vi "test_F9P_fgv-ver.vi"() -> ()   [LabVIEW 2019] (continued)
N,0.221,K,A*35\r\n$GNGGA,065002.00,3723.57089,N,12657.01324,E,1,12,0.74,36.5,M,18.5,M,,*7A\r\n$GNGSA,A,3,17,19,06,12,05,02,09,,,,,,1.34,0.74,1.12,1*03\r\n$GNGSA,A,3,85,71,72,,,,,,,,,,1.34,0.74,1.12,2*0B\r\n$GNGSA,A,3,36,11,04,09,12,,,,,,,,1.34,0.74,1.12,3*0F\r\n$GNGSA,A,3,28,11,14,13,33,08,10,,,,,,1.34,0.74,1.12,4*07\r\n$GPGSV,4,1,13,02,67,338,32,04,06,036,14,05,50,265,42,06,56,081,36,1*65\r\n$GPGSV,4,2,13,07,08,102,,09,36,055,32,12,17,260,32,13,11,191,26,1*6E\r\n$GPGSV,4,3,13,17,16,158,36,19,34,162,29,25,11,291,25,29,09,322,26,1*67\r\n$GPGSV,4,4,13,30,03,132,,1*56\r\n$GPGSV,4,1,13,02,67,338,,04,06,036,,05,50,265,32,06,56,081,30,6*67\r\n$GPGSV,4,2,13,07,08,102,,09,36,055,39,12,17,260,20,13,11,191,,6*65\r\n$GPGSV,4,3,13,17,16,158,34,19,34,162,,25,11,291,20,29,09,322,26,6*6C\r\n$GPGSV,4,4,13,30,03,132,,6*51\r\n$GLGSV,2,1,06,70,51,030,,71,72,230,37,72,20,218,41,84,06,136,10,1*7D\r\n$GLGSV,2,2,06,85,61,118,37,86,55,338,,1*7E\r\n$GLGSV,2,1,06,70,51,030,,71,72,230,26,72,20,218,26,84,06,136,07,3*78\r\n$GLGSV,2,2,06,85,61,118,25,86,55,338,,3*7F\r\n$GAGSV,3,1,09,02,03,285,10,04,67,079,31,05,00,212,,09,47,197,38,7*74\r\n$GAGSV,3,2,09,11,78,050,27,12,30,117,31,18,58,277,45,19,15,041,,7*7F\r\n$GAGSV,3,3,09,36,37,315,22,7*4C\r\n$GAGSV,3,1,09,02,03,285,,04,67,079,34,05,00,212,,09,47,197,36,2*7B\r\n$GAGSV,3,2,09,11,78,050,27,12,30,117,31,18,58,277,35,19,15,041,,2*7D\r\n$GAGSV,3,3,09,36,37,315,34,2*4E\r\n$GBGSV,5,1,17,01,42,153,,03,45,207,,04,35,133,,05,09,257,,1*7C\r\n$GBGSV,5,2,17,06,29,183,,07,08,201,,08,66,357,29,09,08,194,,1*73\r\n$GBGSV,5,3,17,10,14,222,26,11,34,144,26,13,50,316,32,14,73,036,35,1*76\r\n$GBGSV,5,4,17,16,25,186,34,27,10,317,,28,61,307,30,33,75,247,37,1*75\r\n$GBGSV,5,5,17,34,10,143,,1*40\r\n$GBGSV,5,1,17,01,42,153,,03,45,207,,04,35,133,,05,09,257,,3*7E\r\n$GBGSV,5,2,17,06,29,183,,07,08,201,,08,66,357,21,09,08,194,,3*79\r\n$GBGSV,5,3,17,10,14,222,39,11,34,144,39,13,50,316,24,14,73,036,29,3*7E\r\n$GBGSV,5,4,17,16,25,186,33,27,10,317,,28,61,307,,33,75,247,,3*77\r\n$GBGSV,5,5,17,34,10,143,,3*42\r\n$GNGLL,3723.57089,N,12657.01324,E,065002.00,A,A*73\r\n$GNRMC,065003.00,A,3723.57090,N,12657.01323,E,0.098,,250720,,,A,V*1D\r\n$GNVTG,,T,,M,0.098,N,0.182,K,A*37\r\n$GNGGA,065003.00,3723.57090,N,12657.01323,E,1,12,0.74,36.5,M,18.5,M,,*74\r\n$GNGSA,A,3,17,19,06,12,05,02,09,,,,,,1.34,0.74,1.12,1*03\r\n$GNGSA,A,3,85,71,72,,,,,,,,,,1.34,0.74,1.12,2*0B\r\n$GNGSA,A,3,36,11,04,09,12,,,,,,,,1.34,0.74,1.12,3*0F\r\n$GNGSA,A,3,28,11,14,13,33,08,10,,,,,,1.34,0.74,1.12,4*07\r\n$GPGSV,4,1,13,02,67,338,34,04,06,036,09,05,50,265,43,06,56,081,33,1*6B\r\n$GPGSV,4,2,13,07,08,102,14,09,36,055,31,12,17,260,25,13,11,191,27,1*6F\r\n$GPGSV,4,3,13,17,16,158,35,19,34,162,27,25,11,291,20,29,09,322,23,1*6A\r\n$GPGSV,4,4,13,30,03,132,,1*56\r\n$GPGSV,4,1,13,02,67,338,,04,06,036,,05,50,265,32,06,56,081,21,6*67\r\n$GPGSV,4,2,13,07,08,102,,09,36,055,38,12,17,260,20,13,11,191,,6*64\r\n$GPGSV,4,3,13,17,16,158,36,19,34,162,,25,11,291,19,29,09,322,25,6*67\r\n$GPGSV,4,4,13,30,03,132,,6*51\r\n$GLGSV,2,1,06,70,51,030,,71,72,230,40,72,20,218,40,84,06,136,11,1*7D\r\n$GLGSV,2,2,06,85,61,118,37,86,55,338,,1*7E\r\n$GLGSV,2,1,06,70,51,030,,71,72,230,23,72,20,218,27,84,06,136,08,3*73\r\n$GLGSV,2,2,06,85,61,118,23,86,55,338,,3*79\r\n$GAGSV,3,1,09,02,03,285,08,04,67,079,25,05,00,212,,09,47,197,37,7*77\r\n$GAGSV,3,2,09,11,78,050,27,12,30,117,30,18,58,277,44,19,15,041,19,7*77\r\n$GAGSV,3,3,09,36,37,315,17,7*4A\r\n$GAGSV,3,1,09,02,03,285,,04,67,079,30,05,00,212,,09,47,197,33,2*7A\r\n$GAGSV,3,2,09,11,78,050,23,12,30,117,29,18,58,277,32,19,15,041,,2*77\r\n$GAGSV,3,3,09,36,37,315,34,2*4E\r\n$GBGSV,5,1,17,01,42,153,,03,45,207,,04,35,133,,05,09,257,,1*7C\r\n$GBGSV,5,2,17,06,29,183,,07,08,201,,08,66,357,28,09,08,194,,1*72\r\n$GBGSV,5,3,17,10,14,222,25,11,34,144,30,13,50,316,25,14,73,036,34,1*75\r\n$GBGSV,5,4,17,16,25,186,31,27,10,317,,28,61,307,30,33,75,247,39,1*7E\r\n$GBGSV,5,5,17,34,10,143,,1*40\r\n$GBGSV,5,1,17,01,42,153,,03,45,207,,04,35,133,,05,09,257,,3*7E\r\n$GBGSV,5,2,17,06,29,183,,07,08,201,,08,66,357,21,09,08,194,,3*79\r\n$GBGSV,5,3,17,10,14,222,39,11,34,144,41,13,50,316,25,14,73,036,28,3*71\r\n$GBGSV,5,4,17,16,25,186,33,27,10,317,,28,61,307,,33,75,247,,3*77\r\n$GBGSV,5,5,17,34,10,143,,3*42\r\n$GNGLL,3723.57090,N,12657.01323,E,065003.00,A,A*7D\r\n$GNRMC,065004.00,A,3723.57091,N,12657.01321,E,0.157,,250720,,,A,V*1B\r\n$GNVTG,,T,,M,0.157,N,0.291,K,A*34\r\n$GNGGA,065004.00,3723.57091,N,12657.01321,E,1,12,0.71,36.5,M,18.5,M,,*75\r\n$GNGSA,A,3,17,19,06,12,05,02,09,,,,,,1.26,0.71,1.04,1*02\r\n$GNGSA,A,3,85,71,72,,,,,,,,,,1.26,0.71,1.04,2*0A\r\n$GNGSA,A,3,36,11,04,09,12,,,,,,,,1.26,0.71,1.04,3*0E\r\n$GNGSA,A,3,28,11,14,13,33,08,10,,,,,,1.26,0.71,1.04,4*06\r\n$GPGSV,4,1,13,02,67,338,23,04,06,036,09,05,50,265,42,06,56,081,29,1*67\r\n$GPGSV,4,2,13,07,08,102,11,09,36,055,33,12,17,260,26,13,11,191,28,1*64\r\n$GPGSV,4,3,13,17,16,158,43,19,34,162,35,25,11,291,21,29,09,322,25,1*6F\r\n$GPGSV,4,4,13,30,03,132,,1*56\r\n$GPGSV,4,1,13,02,67,338,,04,06,036,,05,50,265,30,06,56,081,25,6*61\r\n$GPGSV,4,2,13,07,08,102,,09,36,055,37,12,17,260,20,13,11,191,,6*6B\r\n$GPGSV,4,3,13,17,16,158,32,19,34,162,,25,11,291,17,29,09,322,24,6*6C\r\n$GPGSV,4,4,13,30,03,132,,6*51\r\n$GLGSV,2,1,06,70,50,030,,71,72,230,41,72,20,218,36,84,06,136,12,1*7F\r\n$GLGSV,2,2,06,85,61,118,33,86,55,338,,1*7A\r\n$GLGSV,2,1,06,70,50,030,,71,72,230,18,72,20,218,26,84,06,136,10,3*72\r\n$GLGSV,2,2,06,85,61,118,34,86,55,338,,3*7F\r\n$GAGSV,3,1,09,02,03,285,09,04,67,079,27,05,00,212,,09,47,197,31,7*72\r\n$GAGSV,3,2,09,11,78,050,29,12,30,117,30,18,58,277,40,19,15,041,15,7*71\r\n$GAGSV,3,3,09,36,37,315,14,7*49\r\n$GAGSV,3,1,09,02,03,285,,04,67,079,30,05,00,212,,09,47,197,34,2*7D\r\n$GAGSV,3,2,09,11,78,050,20,12,30,117,29,18,58,277,27,19,15,041,,2*70\r\n$GAGSV,3,3,09,36,37,315,38,2*42\r\n$GBGSV,5,1,17,01,42,153,,03,45,207,,04,35,133,,05,09,257,,1*7C\r\n$GBGSV,5,2,17,06,29,183,,07,08,201,,08,66,357,18,09,08,194,,1*71\r\n$GBGSV,5,3,17,10,14,222,32,11,34,144,21,13,50,316,24,14,73,036,34,1*72\r\n$GBGSV,5,4,17,16,25,186,30,27,10,317,,28,61,307,30,33,75,247,39,1*7F\r\n$GBGSV,5,5,17,34,10,143,,1*40\r\n$GBGSV,5,1,17,01,42,153,,03,45,207,,04,35,133,,05,09,257,,3*7E\r\n$GBGSV,5,2,17,06,29,183,,07,08,201,,08,66,357,18,09,08,194,,3*73\r\n$GBGSV,5,3,17,10,14,222,34,11,34,144,40,13,50,316,24,14,73,036,26,3*72\r\n$GBGSV,5,4,17,16,25,186,32,27,10,317,,28,61,307,,33,75,247,,3*76\r\n$GBGSV,5,5,17,34,10,143,,3*42\r\n$GNGLL,3723.57091,N,12657.01321,E,065004.00,A,A*79\r\n$GNRMC,065005.00,A,3723.57095,N,12657.01320,E,0.067,,250720,,,A,V*1D\r\n$GNVTG,,T,,M,0.067,N,0.125,K,A*3A\r\n$GNGGA,065005.00,3723.57095,N,12657.01320,E,1,12,0.85,36.4,M,18.5,M,,*7B\r\n$GNGSA,A,3,17,19,06,12,05,02,09,,,,,,1.53,0.85,1.27,1*0A\r\n$GNGSA,A,3,85,71,72,,,,,,,,,,1.53,0.85,1.27,2*02\r\n$GNGSA,A,3,36,11,04,09,12,,,,,,,,1.53,0.85,1.27,3*06\r\n$GNGSA,A,3,28,11,14,13,33,08,10,,,,,,1.53,0.85,1.27,4*0E\r\n$GPGSV,4,1,13,02,67,338,23,04,06,036,15,05,50,265,41,06,56,081,27,1*67\r\n$GPGSV,4,2,13,07,08,102,,09,36,055,34,12,17,260,25,13,11,191,26,1*6E\r\n$GPGSV,4,3,13,17,16,158,45,19,34,162,32,25,11,291,22,29,09,322,25,1*6D\r\n$GPGSV,4,4,13,30,03,132,,1*56\r\n$GPGSV,4,1,13,02,67,338,,04,06,036,,05,50,265,22,06,56,081,30,6*66\r\n$GPGSV,4,2,13,07,08,102,,09,36,055,37,12,17,260,22,13,11,191,,6*69\r\n$GPGSV,4,3,13,17,16,158,35,19,34,162,,25,11,291,16,29,09,322,25,6*6B\r\n$GPGSV,4,4,13,30,03,132,,6*51\r\n$GLGSV,2,1,06,70,50,030,,71,72,232,40,72,20,218,36,84,06,136,08,1*77\r\n$GLGSV,2,2,06,85,61,118,32,86,55,338,,1*7B\r\n$GLGSV,2,1,06,70,50,030,,71,72,232,27,72,20,218,27,84,06,136,10,3*7D\r\n$GLGSV,2,2,06,85,61,118,34,86,55,338,,3*7F\r\n$GAGSV,3,1,09,02,03,285,08,04,67,079,33,05,00,212,,09,47,197,27,7*71\r\n$GAGSV,3,2,09,11,78,050,32,12,30,117,29,18,58,277,41,19,15,041,10,7*77\r\n$GAGSV,3,3,09,36,37,315,11,7*4C\r\n$GAGSV,3,1,09,02,03,285,,04,67,079,28,05,00,212,,09,47,197,34,2*74\r\n$GAGSV,3,2,09,11,78,050,14,12,30,117,29,18,58,277,35,19,15,041,,2*74\r\n$GAGSV,3,3,09,36,37,315,39,2*43\r\n$GBGSV,5,1,17,01,42,153,,03,45,207,,04,35,133,,05,09,257,,1*7C\r\n$GBGSV,5,2,17,06,29,183,,07,08,201,,08,66,357,17,09,08,194,,1*7E\r\n$GBGSV,5,3,17,10,14,222,32,11,34,144,22,13,50,316,22,14,73,036,33,1*70\r\n$GBGSV,5,4,17,16,25,186,34,27,10,317,,28,61,307,30,33,75,247,36,1*74\r\n$GBGSV,5,5,17,34,10,143,,1*40\r\n$GBGSV,5,1,17,01,42,153,,03,45,207,,04,35,133,,05,09,257,,3*7E\r\n$GBGSV,5,2,17,06,29,183,,07,08,201,,08,66,357,19,09,08,194,,3*72\r\n$GBGSV,5,3,17,10,14,222,29,11,34,144,35,13,50,316,27,14,73,036,24,3*7D\r\n$GBGSV,5,4,17,16,25,186,31,27,10,317,,28,61,307,,33,75,247,,3*75\r\n$GBGSV,5,5,17,34,10,143,,3*42\r\n$GNGLL,3723.57095,N,12657.01320,E,065005.00,A,A*7D\r\n$GNRMC,065006.00,A,3723.57082,N,12657.01322,E,0.705,187.77,250720,,,A,V*09\r\n$GNVTG,187.77,T,,M,0.705,N,1.305,K,A*28\r\n$GNGGA,065006.00,3723.57082,N,12657.01322,E,1,12,0.74,36.4,M,18.5,M,,*72\r\n$GNGSA,A,3,17,19,06,12,05,02,09,,,,,,1.34,0.74,1.12,1*03\r\n$GNGSA,A,3,85,71,72,,,,,,,,,,1.34,0.74,1.12,2*0B\r\n$GNGSA,A,3,36,19,11,04,09,12,,,,,,,1.34,0.74,1.12,3*07\r\n$GNGSA,A,3,28,11,14,13,33,08,10,,,,,,1.34,0.74,1.12,4*07\r\n$GPGSV,4,1,13,02,67,338,31,04,06,036,07,05,50,265,45,06,56,081,40,1*62\r\n$GPGSV,4,2,13,07,08,102,,09,36,055,33,12,17,260,25,13,11,191,24,1*6B\r\n$GPGSV,4,3,13,17,16,158,36,19,34,162,42,25,11,291,30,29,09,322,31,1*68\r\n$GPGSV,4,4,13,30,03,132,,1*56\r\n$GPGSV,4,1,13,02,67,338,,04,06,036,,05,50,265,31,06,56,081,35,6*61\r\n$GPGSV,4,2,13,07,08,102,,09,36,055,34,12,17,260,22,13,11,191,,6*6A\r\n$GPGSV,4,3,13,17,16,158,27,19,34,162,,25,11,291,16,29,09,322,27,6*6A\r\n$GPGSV,4,4,13,30,03,132,,6*51\r\n$GLGSV,2,1,06,70,50,030,,71,72,232,40,72,21,219,47,84,06,136,08,1*71\r\n$GLGSV,2,2,06,85,61,118,42,86,55,338,,1*7C\r\n$GLGSV,2,1,06,70,50,030,,71,72,232,25,72,21,219,37,84,06,136,11,3*7F\r\n$GLGSV,2,2,06,85,61,118,29,86,55,338,,3*73\r\n$GAGSV,3,1,09,02,03,285,08,04,67,079,39,05,00,212,,09,47,197,40,7*7A\r\n$GAGSV,3,2,09,11,78,050,36,12,30,117,29,18,58,277,48,19,15,041,08,7*73\r\n$GAGSV,3,3,09,36,37,315,21,7*4F\r\n$GAGSV,3,1,09,02,03,285,,04,67,079,37,05,00,212,,09,47,197,37,2*79\r\n$GAGSV,3,2,09,11,78,050,27,12,30,117,29,18,58,277,41,19,15,041,,2*77\r\n$GAGSV,3,3,09,36,37,315,32,2*48\r\n$GBGSV,5,1,17,01,42,153,,03,45,207,,04,35,133,,05,09,257,,1*7C\r\n$GBGSV,5,2,17,06,29,183,,07,08,201,,08,66,357,20,09,08,194,,1*7A\r\n$GBGSV,5,3,17,10,14,222,44,11,34,144,39,13,50,316,30,14,73,036,38,1*73\r\n$GBGSV,5,4,17,16,25,186,41,27,10,317,,28,61,307,34,33,75,247,45,1*76\r\n$GBGSV,5,5,17,34,10,143,,1*40\r\n$GBGSV,5,1,17,01,42,153,,03,45,207,,04,35,133,,05,09,257,,3*7E\r\n$GBGSV,5,2,17,06,29,183,,07,08,201,,08,66,357,24,09,08,194,,3*7C\r\n$GBGSV,5,3,17,10,14,222,32,11,34,144,45,13,50,316,28,14,73,036,30,3*7A\r\n$GBGSV,5,4,17,16,25,186,27,27,10,317,,28,61,307,,33,75,247,,3*72\r\n$GBGSV,5,5,17,34,10,143,,3*42\r\n$GNGLL,3723.57082,N,12657.01322,E,065006.00,A,A*7A\r\n$GNRMC,065007.00,A,3723.57072,N,12657.01317,E,0.309,,250720,,,A,V*19\r\n$GNVTG,,T,,M,0.309,N,0.572,K,A*37\r\n$GNGGA,065007.00,3723.57072,N,12657.01317,E,1,12,0.74,36.5,M,18.5,M,,*7B\r\n$GNGSA,A,3,17,19,06,12,05,02,09,,,,,,1.34,0.74,1.12,1*03\r\n$GNGSA,A,3,85,71,72,,,,,,,,,,1.34,0.74,1.12,2*0B\r\n$GNGSA,A,3,36,19,11,04,09,12,,,,,,,1.34,0.74,1.12,3*07\r\n$GNGSA,A,3,28,11,14,13,33,08,10,,,,,,1.34,0.74,1.12,4*07\r\n$GPGSV,4,1,13,02,67,338,36,04,06,036,20,05,50,265,41,06,56,081,43,1*67\r\n$GPGSV,4,2,13,07,08,102,,09,36,055,38,12,17,260,24,13,11,191,,1*67\r\n$GPGSV,4,3,13,17,16,158,41,19,34,162,42,25,11,291,29,29,09,322,35,1*64\r\n$GPGSV,4,4,13,30,03,132,,1*56\r\n$GPGSV,4,1,13,02,67,338,,04,06,036,,05,50,265,35,06,56,081,36,6*66\r\n$GPGSV,4,2,13,07,08,102,,09,36,055,31,12,17,260,26,13,11,191,,6*6B\r\n$GPGSV,4,3,13,17,16,158,19,19,34,162,,25,11,291,23,29,09,322,27,6*61\r\n$GPGSV,4,4,13,30,03,132,,6*51\r\n$GLGSV,2,1,06,70,50,030,,71,72,232,45,72,21,219,39,84,06,136,11,1*75\r\n$GLGSV,2,2,06,85,61,118,44,86,55,338,,1*7A\r\n$GLGSV,2,1,06,70,50,030,,71,72,232,25,72,21,219,39,84,06,136,06,3*77\r\n$GLGSV,2,2,06,85,61,118,35,86,55,338,,3*7E\r\n$GAGSV,3,1,09,02,03,285,11,04,67,079,40,05,00,212,,09,47,197,41,7*7D\r\n$GAGSV,3,2,09,11,78,050,35,12,30,117,34,18,58,277,46,19,15,041,14,7*7F\r\n$GAGSV,3,3,09,36,37,315,16,7*4B\r\n$GAGSV,3,1,09,02,03,285,,04,67,079,37,05,00,212,,09,47,197,39,2*77\r\n$GAGSV,3,2,09,11,78,050,33,12,30,117,34,18,58,277,38,19,15,041,,2*70\r\n$GAGSV,3,3,09,36,37,315,33,2*49\r\n$GBGSV,5,1,17,01,42,153,,03,45,207,,04,35,133,,05,09,257,,1*7C\r\n$GBGSV,5,2,17,06,29,183,,07,08,201,,08,66,357,23,09,08,194,,1*79\r\n$GBGSV,5,3,17,10,14,222,35,11,34,144,40,13,50,316,23,14,73,036,31,1*70\r\n$GBGSV,5,4,17,16,25,186,28,27,10,317,,28,61,307,25,33,75,247,41,1*7D\r\n$GBGSV,5,5,17,34,10,143,,1*40\r\n$GBGSV,5,1,17,01,42,153,,03,45,207,,04,35,133,,05,09,257,,3*7E\r\n$GBGSV,5,2,17,06,29,183,,07,08,201,,08,66,357,24,09,08,194,,3*7C\r\n$GBGSV,5,3,17,10,14,222,39,11,34,144,39,13,50,316,28,14,73,036,35,3*7F\r\n$GBGSV,5,4,17,16,25,186,27,27,10,317,,28,61,307,,33,75,247,,3*72\r\n$GBGSV,5,5,17,34,10,143,,3*42\r\n$GNGLL,3723.57072,N,12657.01317,E,065007.00,A,A*72\r\n$GNRMC,065008.00,A,3723.57072,N,12657.01318,E,0.185,,250720,,,A,V*1F\r\n$GNVTG,,T,,M,0.185,N,0.342,K,A*34\r\n$GNGGA,065008.00,3723.57072,N,12657.01318,E,1,12,0.71,36.5,M,18.5,M,,*7E\r\n$GNGSA,A,3,17,19,06,12,05,02,09,,,,,,1.26,0.71,1.04,1*02\r\n$GNGSA,A,3,85,71,72,,,,,,,,,,1.26,0.71,1.04,2*0A\r\n$GNGSA,A,3,36,19,11,04,09,12,,,,,,,1.26,0.71,1.04,3*06\r\n$GNGSA,A,3,28,11,14,13,33,08,10,,,,,,1.26,0.71,1.04,4*06\r\n$GPGSV,4,1,13,02,67,338,37,04,06,036,16,05,50,265,42,06,56,081,44,1*67\r\n$GPGSV,4,2,13,07,08,102,,09,36,055,39,12,17,260,23,13,11,191,25,1*66\r\n$GPGSV,4,3,13,17,16,158,43,19,34,162,43,25,11,291,28,29,09,322,32,1*61\r\n$GPGSV,4,4,13,30,03,132,,1*56\r\n$GPGSV,4,1,13,02,67,338,,04,06,036,,05,50,265,38,06,56,081,38,6*65\r\n$GPGSV,4,2,13,07,08,102,,09,36,055,31,12,17,260,23,13,11,191,,6*6E\r\n$GPGSV,4,3,13,17,16,158,24,19,34,162,,25,11,291,25,29,09,322,27,6*69\r\n$GPGSV,4,4,13,30,03,132,,6*51\r\n$GLGSV,2,1,06,70,50,030,,71,72,232,45,72,21,219,38,84,06,136,10,1*75\r\n$GLGSV,2,2,06,85,61,118,44,86,55,338,,1*7A\r\n$GLGSV,2,1,06,70,50,030,,71,72,232,27,72,21,219,38,84,06,136,08,3*7A\r\n$GLGSV,2,2,06,85,61,118,35,86,55,338,,3*7E\r\n$GAGSV,3,1,09,02,03,285,10,04,67,079,39,05,00,212,,09,47,197,42,7*71\r\n$GAGSV,3,2,09,11,78,050,35,12,30,117,33,18,58,277,46,19,15,041,09,7*74\r\n$GAGSV,3,3,09,36,37,315,29,7*47\r\n$GAGSV,3,1,09,02,03,285,,04,67,079,35,05,00,212,,09,47,197,40,2*7B\r\n$GAGSV,3,2,09,11,78,050,33,12,30,117,35,18,58,277,40,19,15,041,,2*7E\r\n$GAGSV,3,3,09,36,37,315,36,2*4C\r\n$GBGSV,5,1,17,01,42,153,,03,45,207,,04,35,133,,05,09,257,,1*7C\r\n$GBGSV,5,2,17,06,29,183,,07,08,201,,08,66,357,30,09,08,194,,1*7B\r\n$GBGSV,5,3,17,10,14,222,34,11,34,144,41,13,50,316,24,14,73,036,33,1*75\r\n$GBGSV,5,4,17,16,25,186,30,27,10,317,,28,61,307,31,33,75,247,43,1*73\r\n$GBGSV,5,5,17,34,10,143,,1*40\r\n$GBGSV,5,1,17,01,42,153,,03,45,207,,04,35,133,,05,09,257,,3*7E\r\n$GBGSV,5,2,17,06,29,183,,07,08,201,,08,66,357,26,09,08,194,,3*7E\r\n$GBGSV,5,3,17,10,14,222,41,11,34,144,40,13,50,316,28,14,73,036,37,3*7C\r\n$GBGSV,5,4,17,16,25,186,26,27,10,317,,28,61,307,,33,75,247,,3*73\r\n$GBGSV,5,5,17,34,10,143,,3*42\r\n$GNGLL,3723.57072,N,12657.01318,E,065008.00,A,A*72\r\n$GNRMC,065009.00,A,3723.57073,N,12657.01317,E,0.049,,250720,,,A,V*11\r\n$GNVTG,,T,,M,0.049,N,0.090,K,A*39\r\n$GNGGA,065009.00,3723.57073,N,12657.01317,E,1,12,0.65,36.5,M,18.5,M,,*74\r\n$GNGSA,A,3,17,19,06,12,05,02,09,,,,,,1.11,0.65,0.90,1*0F\r\n$GNGSA,A,3,85,71,72,,,,,,,,,,1.11,0.65,0.90,2*07\r\n$GNGSA,A,3,36,19,11,04,09,12,,,,,,,1.11,0.65,0.90,3*0B\r\n$GNGSA,A,3,28,11,14,13,33,08,10,,,,,,1.11,0.65,0.90,4*0B\r\n$GPGSV,4,1,13,02,67,338,36,04,06,036,18,05,50,265,43,06,56,081,44,1*69\r\n$GPGSV,4,2,13,07,08,102,,09,36,055,41,12,17,260,29,13,11,191,25,1*63\r\n$GPGSV,4,3,13,17,16,158,40,19,34,162,42,25,11,291,29,29,09,322,32,1*62\r\n$GPGSV,4,4,13,30,03,132,,1*56\r\n$GPGSV,4,1,13,02,67,338,,04,06,036,,05,50,265,40,06,56,081,42,6*67\r\n$GPGSV,4,2,13,07,08,102,,09,36,055,35,12,17,260,22,13,11,191,,6*6B\r\n$GPGSV,4,3,13,17,16,158,36,19,34,162,,25,11,291,27,29,09,322,32,6*6C\r\n$GPGSV,4,4,13,30,03,132,,6*51\r\n$GLGSV,2,1,06,70,50,030,,71,72,232,44,72,21,219,32,84,06,136,09,1*76\r\n$GLGSV,2,2,06,85,61,118,42,86,55,338,,1*7C\r\n$GLGSV,2,1,06,70,50,030,,71,72,232,28,72,21,219,39,84,06,136,08,3*74\r\n$GLGSV,2,2,06,85,61,118,36,86,55,338,,3*7D\r\n$GAGSV,3,1,09,02,03,285,10,04,67,079,38,05,00,212,,09,47,197,41,7*73\r\n$GAGSV,3,2,09,11,78,050,35,12,30,117,33,18,58,277,44,19,15,041,16,7*78\r\n$GAGSV,3,3,09,36,37,315,37,7*48\r\n$GAGSV,3,1,09,02,03,285,,04,67,079,36,05,00,212,,09,47,197,40,2*78\r\n$GAGSV,3,2,09,11,78,050,33,12,30,117,35,18,58,277,40,19,15,041,,2*7E\r\n$GAGSV,3,3,09,36,37,315,38,2*42\r\n$GBGSV,5,1,17,01,42,153,,03,45,207,,04,35,133,,05,09,257,,1*7C\r\n$GBGSV,5,2,17,06,29,183,,07,08,201,,08,66,357,31,09,08,194,,1*7A\r\n$GBGSV,5,3,17,10,14,222,36,11,34,144,41,13,50,316,24,14,73,036,36,1*72\r\n$GBGSV,5,4,17,16,25,186,28,27,10,317,,28,61,307,28,33,75,247,43,1*72\r\n$GBGSV,5,5,17,34,10,143,,1*40\r\n$GBGSV,5,1,17,01,42,153,,03,45,207,,04,35,133,,05,09,257,,3*7E\r\n$GBGSV,5,2,17,06,29,183,,07,08,201,,08,66,357,25,09,08,194,,3*7D\r\n$GBGSV,5,3,17,10,14,222,41,11,34,144,41,13,50,316,29,14,73,036,38,3*73\r\n$GBGSV,5,4,17,16,25,186,23,27,10,317,,28,61,307,,33,75,247,,3*76\r\n$GBGSV,5,5,17,34,10,143,,3*42\r\n$GNGLL,3723.57073,N,12657.01317,E,065009.00,A,A*7D\r\n$GNRMC,065010.00,A,3723.57074,N,12657.01314,E,0.036,,250720,,,A,V*15\r\n$GNVTG,,T,,M,0.036,N,0.066,K,A*38\r\n$GNGGA,065010.00,3723.57074,N,12657.01314,E,1,12,0.65,36.5,M,18.5,M,,*78\r\n$GNGSA,A,3,17,19,06,12,05,02,09,,,,,,1.11,0.65,0.90,1*0F\r\n$GNGSA,A,3,85,71,72,,,,,,,,,,1.11,0.65,0.90,2*07\r\n$GNGSA,A,3,36,19,11,04,09,12,,,,,,,1.11,0.65,0.90,3*0B\r\n$GNGSA,A,3,28,11,14,13,33,08,10,,,,,,1.11,0.65,0.90,4*0B\r\n$GPGSV,4,1,13,02,67,338,34,04,06,036,19,05,50,265,42,06,56,081,44,1*6B\r\n$GPGSV,4,2,13,07,08,102,,09,36,055,40,12,17,260,29,13,11,191,25,1*62\r\n$GPGSV,4,3,13,17,16,158,40,19,34,162,42,25,11,291,30,29,09,322,27,1*6E\r\n$GPGSV,4,4,13,30,03,132,,1*56\r\n$GPGSV,4,1,13,02,67,338,,04,06,036,20,05,50,265,39,06,56,081,41,6*68\r\n$GPGSV,4,2,13,07,08,102,,09,36,055,34,12,17,260,20,13,11,191,,6*68\r\n$GPGSV,4,3,13,17,16,158,35,19,34,162,,25,11,291,28,29,09,322,31,6*63\r\n$GPGSV,4,4,13,30,03,132,,6*51\r\n$GLGSV,2,1,06,70,50,030,,71,72,232,44,72,21,219,31,84,06,136,07,1*7B\r\n$GLGSV,2,2,06,85,61,118,42,86,55,338,,1*7C\r\n$GLGSV,2,1,06,70,50,030,,71,72,232,28,72,21,219,40,84,06,136,10,3*73\r\n$GLGSV,2,2,06,85,61,118,35,86,55,338,,3*7E\r\n$GAGSV,3,1,09,02,03,285,10,04,67,079,38,05,00,212,,09,47,197,41,7*73\r\n$GAGSV,3,2,09,11,78,050,35,12,30,117,34,18,58,277,45,19,15,041,11,7*79\r\n$GAGSV,3,3,09,36,37,315,37,7*48\r\n$GAGSV,3,1,09,02,03,285,,04,67,079,36,05,00,212,,09,47,197,40,2*78\r\n$GAGSV,3,2,09,11,78,050,34,12,30,117,35,18,58,277,41,19,15,041,,2*78\r\n$GAGSV,3,3,09,36,37,315,38,2*42\r\n$GBGSV,5,1,17,01,42,153,,03,45,207,,04,35,133,,05,09,257,,1*7C\r\n$GBGSV,5,2,17,06,29,183,,07,08,201,,08,66,357,30,09,08,194,,1*7B\r\n$GBGSV,5,3,17,10,14,222,33,11,34,144,39,13,50,316,26,14,73,036,33,1*7F\r\n$GBGSV,5,4,17,16,25,186,27,27,10,317,,28,61,307,26,33,75,247,40,1*70\r\n$GBGSV,5,5,17,34,10,143,,1*40\r\n$GBGSV,5,1,17,01,42,153,,03,45,207,,04,35,133,,05,09,257,,3*7E\r\n$GBGSV,5,2,17,06,29,183,,07,08,201,,08,66,357,25,09,08,194,,3*7D\r\n$GBGSV,5,3,17,10,14,222,42,11,34,144,41,13,50,316,29,14,73,036,38,3*70\r\n$GBGSV,5,4,17,16,25,186,20,27,10,317,,28,61,307,,33,75,247,,3*75\r\n$GBGSV,5,5,17,34,10,143,,3*42\r\n$GNGLL,3723.57074,N,12657.01314,E,065010.00,A,A*71\r\n$GNRMC,065011.00,A,3723.57075,N,12657.01314,E,0.051,,250720,,,A,V*14\r\n$GNVTG,,T,,M,0.051,N,0.095,K,A*35\r\n$GNGGA,065011.00,3723.57075,N,12657.01314,E,1,12,0.71,36.6,M,18.5,M,,*7E\r\n$GNGSA,A,3,17,19,06,12,05,02,09,,,,,,1.26,0.71,1.04,1*02\r\n$GNGSA,A,3,85,71,72,,,,,,,,,,1.26,0.71,1.04,2*0A\r\n$GNGSA,A,3,36,11,04,09,12,,,,,,,,1.26,0.71,1.04,3*0E\r\n$GNGSA,A,3,28,11,14,13,33,08,10,,,,,,1.26,0.71,1.04,4*06\r\n$GPGSV,4,1,13,02,67,
